vi "String2KeyValue.vi"(11 "健值对字符串":string) -> (2 "值数组":string[](array[string]), 3 "键数组":string[](array[string]))   [LabVIEW 2020, in "Curve Editor.lvlib" / "Key Value.lvlib"]
uses:
  Key Value.lvlib
panel:
  # "将键值串拆分为键数组和值数组"
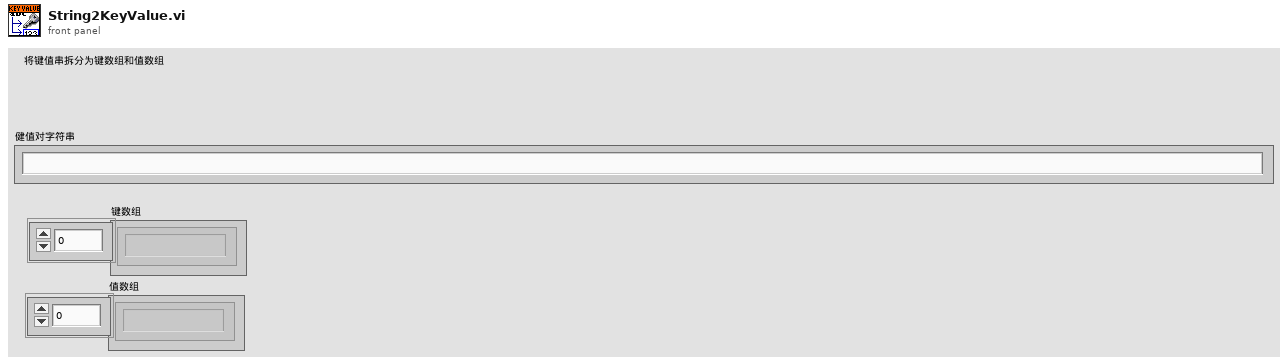
[diagram p1: front panel]
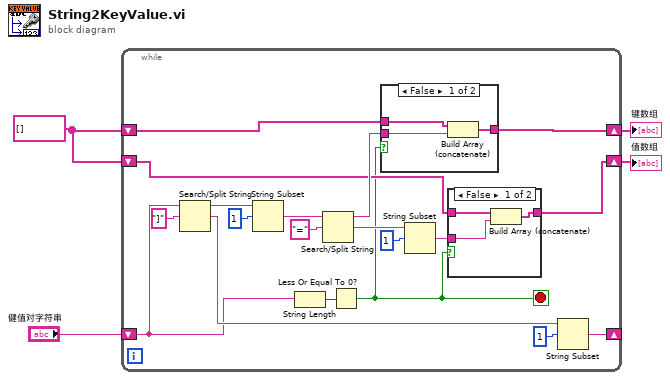
[diagram p0: block diagram]
diagram:
  w4 = string[] []
  n1 = while {
    shift-right: [w18] -> _
    shift-left: "健值对字符串" -> [w17]
    shift-right: [w9] -> w3
    shift-left: w4 -> [w10]
    shift-right: [w7] -> w2
    shift-left: w4 -> [w8]
    stop <- w6 stop-if-true
    n2 = Search/Split String(string=w17, search string/char (-)="]") -> (substring before match=w22:string, match + rest of string=w19:string)  [unwired: 1 in, 1 out]
    n3 = String Subset(string=w22, offset (0)=1 ("偏移量(0)")) -> (substring=w16:string)  [unwired: 1 in]
    n4 = String Length(string=w17) -> (length=w12:i32)
    n5 = Search/Split String(string=w16, search string/char (-)="=" ("子字符串")) -> (substring before match=w11:string, match + rest of string=w14:string)  [unwired: 1 in, 1 out]
    n6 = Less Or Equal To 0?(x=w12) -> (x <= 0?=w6:bool)
    n7 = case shown="False" w6 {
      tunnel: w11 -> [w30 _]
      tunnel: w10 -> [w29 w31]
      tunnel: [w28 w31] -> w9
      frame False {
        n8 = Build Array (concatenate)(w29, w30) -> (w28:string[])
      }
      frame True {
      }
    }
    n9 = String Subset(string=w14, offset (0)=1 ("偏移量(0)")) -> (substring=w5:string)  [unwired: 1 in]
    n10 = case shown="False" w6 {
      tunnel: w5 -> [w26 _]
      tunnel: w8 -> [w25 w27]
      tunnel: [w24 w27] -> w7
      frame False {
        n11 = Build Array (concatenate)(w25, w26) -> (w24:string[])
      }
      frame True {
      }
    }
    n12 = String Subset(string=w19, offset (0)=1 ("偏移量(0)")) -> (substring=w18:string)  [unwired: 1 in]
  }
  "键数组" <- w3
  "值数组" <- w2
